vi "Init MDF.vi"() -> (3 "MDF-Out":T1)   [LabVIEW 2014]
uses:
  MDF.ctl
panel:
  # "Initializes the Mission Definition File"
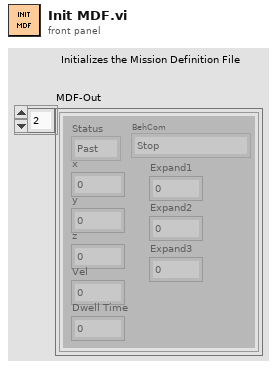
[diagram p1: front panel]
types:
  T1 = typedef "MDF.ctl" = cluster{"Status":enum16{"Past", "Current", "Future"}, "x":dbl, "y":dbl, "z":dbl, "Vel":dbl, "Dwell Time":dbl, "BehCom":enum16{"Stop", "GoToWayPoint", "RightWallFollow", "LeftWallFolllow", "LaneFollow", "CirclePoint"}, "Expand1":dbl, "Expand2":dbl, "Expand3":dbl}[]
  T2 = cluster{"Status":enum16{"Past", "Current", "Future"}, "x":dbl, "y":dbl, "z":dbl, "Vel":dbl, "Dwell Time":dbl, "BehCom":enum16{"Stop", "GoToWayPoint", "RightWallFollow", "LeftWallFolllow", "LaneFollow", "CirclePoint"}, "Expand1":dbl, "Expand2":dbl, "Expand3":dbl}
  T3 = cluster{"Status":enum16{"Past", "Current", "Future"}, "x":dbl, "y":dbl, "z":dbl, "Vel":dbl, "Dwell Time":dbl, "BehCom":enum16{"Stop", "GoToWayPoint", "RightWallFollow", "LeftWallFolllow", "LaneFollow", "CirclePoint"}, "Expand1":dbl, "Expand2":dbl, "Expand3":dbl}[]
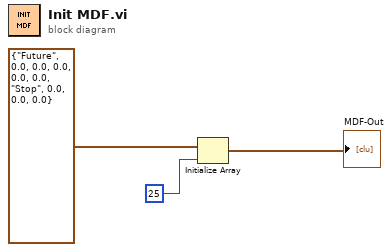
[diagram p0: block diagram]
diagram:
  n1 = Initialize Array "Initialize Array"(T2 {"Status"=enum."Future", "x"=0.0, "y"=0.0, "z"=0.0, "Vel"=0.0, "Dwell Time"=0.0, "BehCom"=enum."Stop", "Expand1"=0.0, "Expand2"=0.0, "Expand3"=0.0} ("new element/subarray"), 25 ("dimension size")) -> (→"MDF-Out":T3)
